vi "Convert String Type Subset.vi"(4 "dst byte order":T3(ring), 5 "src channel descriptor":T1 {"buffer offset" format="%d bytes"}, 6 "src byte order":T3(ring), 7 "dst channel descriptor":T1 {"buffer offset" format="%d bytes"}, 8 "error in (no error)":errorcluster, 9 "channel count":u64, 10 "dst buffer in":string, 11 "src buffer in":string) -> (0 "error out":errorcluster, 2 "dst buffer out":string, 3 "src buffer out":string)   [LabVIEW 2019, in "DSF Core.lvlib" / "Buffer Converter.lvclass"]
uses:
  Buffer Converter.lvclass
  Channel Descriptor.ctl
  Typedefs/DSF Data Type.ctl
  Framework/Framework.lvclass
  DSF Core.lvlib
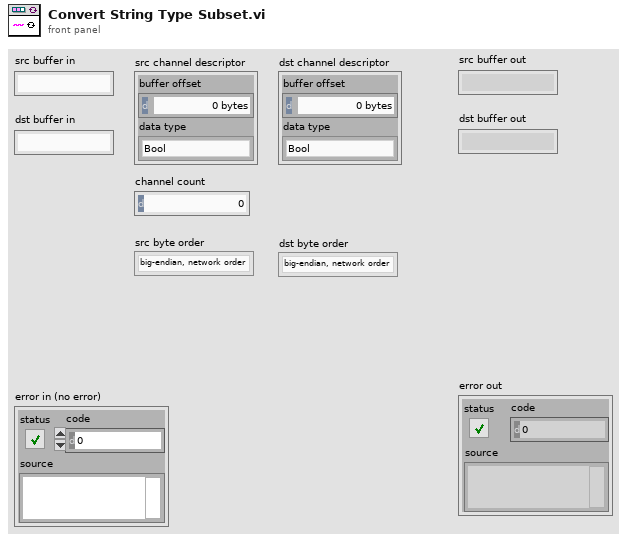
[diagram p1: front panel]
types:
  T1 = typedef "DSF Core.lvlib/Buffer Converter.lvclass/Channel Descriptor.ctl" = cluster{"buffer offset":u64, "data type":T2}
  T2 = typedef "DSF Core.lvlib/DSF Data Type.ctl" = enum8{"Bool", "SGL", "DBL", "I8", "I16", "I32", "I64", "U8", "U16", "U32", "U64"}
  T3 = enum16{"big-endian, network order", "native, host order", "little-endian"}
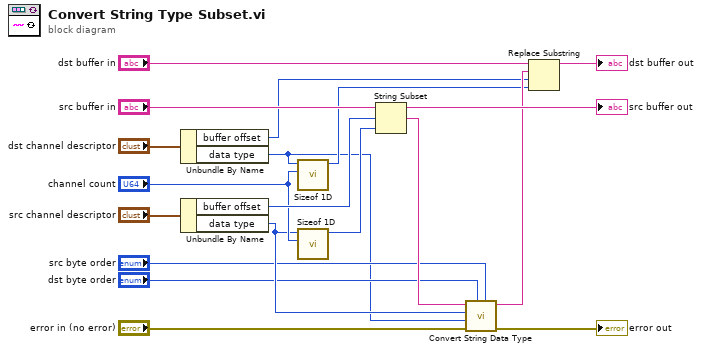
[diagram p0: block diagram]
diagram:
  n1 = Unbundle By Name("dst channel descriptor") -> ("buffer offset"=w5:u64, "data type"=w1:T2)
  n2 = Unbundle By Name("src channel descriptor") -> ("buffer offset"=w13:u64, "data type"=w8:T2)
  n3 = call "Sizeof 1D.vi"("count"="channel count", "data type"=w1) -> ("size in bytes"=w6:u64)  [unwired: 9 in]
  n4 = call "Sizeof 1D.vi"("count"="channel count", "data type"=w8) -> ("size in bytes"=w12:u64)  [unwired: 9 in]
  n5 = String Subset(string="src buffer in", offset (0)=w13, length (rest)=w12) -> (substring=w4:string)
  n6 = call "Convert String Data Type.vi"("src byte order"="src byte order", "dst byte order"="dst byte order", "error in (no error)"="error in (no error)", "dst data type"=w1, "src data type"=w8, "src data in"=w4) -> ("error out"=→"error out":errorcluster, "dst data out"=w7:string)  [unwired: 4 in]
  n7 = Replace Substring(2:w6, 3:w5, 4:w7, 5:"dst buffer in") -> (1:→"dst buffer out":string)  [unwired: 1 out]
  "src buffer out" <- "src buffer in"
